vi "lm Color Level.vi"(8 "error in (no error)":errorcluster, 10 "str_Level":string, 11 "str_Color":string) -> (0 "error out":errorcluster, 2 "str_Level out":string, 3 "str_Color out":string)   [LabVIEW 2017, in "LumencorDLLDbg64.lvlib"]
doc: "Sets the Selected Colors Level.\n\n\nextern \"C\" LUMENCORDLL2B_API void lmColorLevel(char *str_Color, char *str_Level);"
uses:
  LumencorDLLDbg64.lvlib
  LumencorDLLDbg64.dll
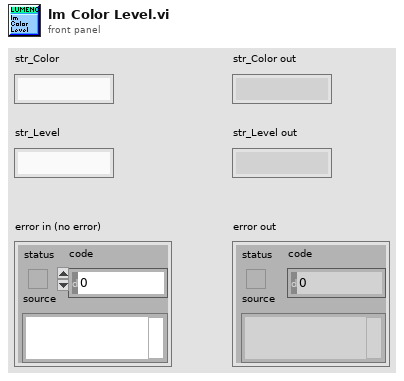
[diagram p1: front panel]
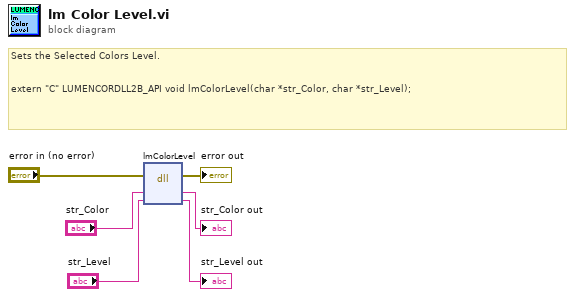
[diagram p0: block diagram]
diagram:
  # "Sets the Selected Colors Level.\n\n\nextern \"C\" LUMENCORDLL2B_API void lmColorLevel(char *str_Color, char *str_Level);"
  n1 = dll-call lib="Q:/GIT -- Lumencor DLL4/LabVIEW Library (64bit)/LumencorDLLDbg64.*" fn="lmColorLevel"(error in="error in (no error)", "str_Color"="str_Color", "str_Level"="str_Level") -> (error out=→"error out":errorcluster, "str_Color"=→"str_Color out":string, "str_Level"=→"str_Level out":string)  [unwired: 3 in, 1 out]
